vi "Process.vi"(8 "error in (no error)":errorcluster, 10 "Wash Step Cycle Completion in":refnum<class "Wash Step Cycle Completion.lvclass">, 11 "Architecture.lvlib:Thread.lvclass":refnum<class "Thread.lvclass">) -> (0 "error out":errorcluster, 1 "Stop?":bool, 3 "Architecture.lvlib:Thread.lvclass 2":refnum<class "Thread.lvclass">)   [LabVIEW 2013, in "Car Wash Controller.lvlib" / "Wash Step Cycle Completion.lvclass"]
uses:
  Wash Step Cycle Completion.lvclass
  Message.lvclass
  Thread.lvclass
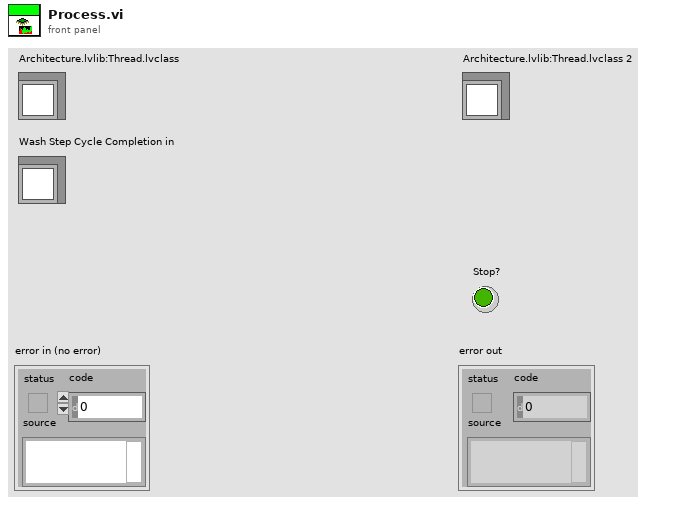
[diagram p1: front panel]
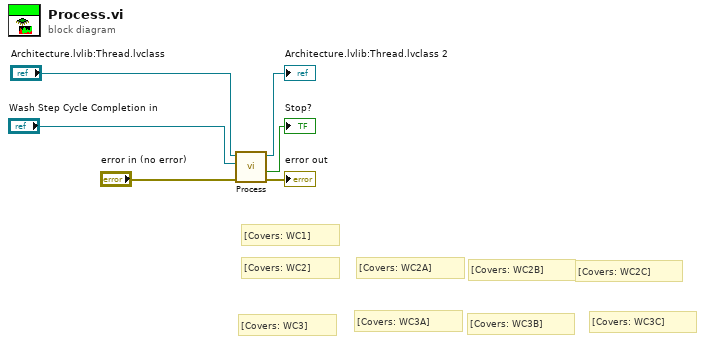
[diagram p0: block diagram]
diagram:
  # "[Covers: WC3C]"
  # "[Covers: WC3B]"
  # "[Covers: WC3A]"
  # "[Covers: WC2C]"
  # "[Covers: WC2B]"
  # "[Covers: WC2A]"
  # "[Covers: WC3]"
  # "[Covers: WC2]"
  # "[Covers: WC1]"
  n1 = call-parent "Process.vi"("error in (no error)"="error in (no error)", "Message in"="Wash Step Cycle Completion in", "Architecture.lvlib:Thread.lvclass"="Architecture.lvlib:Thread.lvclass") -> ("error out"=→"error out":errorcluster, "Stop?"=→"Stop?":bool, "Architecture.lvlib:Thread.lvclass 2"=→"Architecture.lvlib:Thread.lvclass 2":refnum<class "Thread.lvclass">)  [unwired: 6 in]
